vi "Get state -- subVI.vi"(7 "Instrument Channel":string, 8 "error in (no error)":errorcluster, 10 "Address":u8, 11 "Device state in":T2=enum."Configuration") -> (0 "error out":errorcluster, 2 "Controller state":T1, 3 "Device state out":T2)   [LabVIEW 2020, in "FCR100.lvlib"]
uses:
  FCR100.lvlib
  Device state -- enum.ctl
  Controller state -- enum.ctl
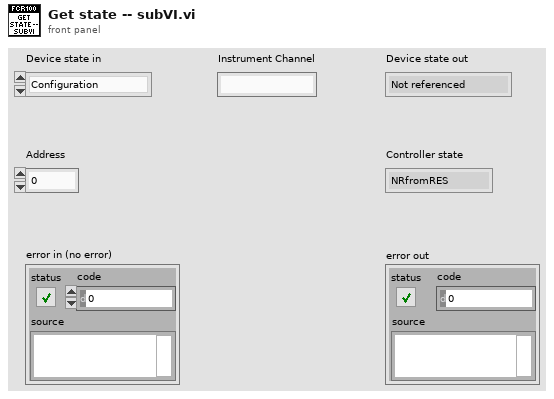
[diagram p1: front panel]
types:
  T1 = typedef "FCR100.lvlib/Controller state -- enum.ctl" = enum16{"NRfromRES", "NRfromHOM", "NRfromCONF", "NRfromDIS", "NRfromRDY", "NRfromMOV", "NR-NPM", "CONFIG", "HOMING", "MOVING", "RDYfromHOM", "RDYfromMOV", "RDYfromDIS", "DISfromRDY", "DISfromMOV"}
  T2 = typedef "FCR100.lvlib/Device state -- enum.ctl" = enum16{"Not referenced", "Configuration", "Disable", "Ready", "Homing", "Motion"}
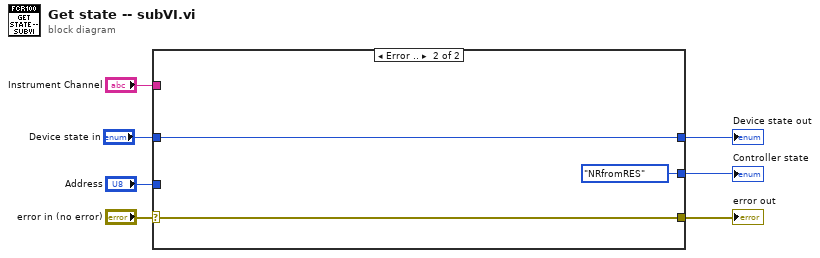
[diagram p0: block diagram]
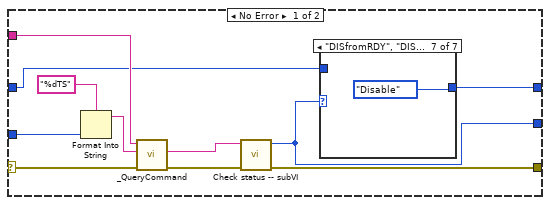
[diagram p2: hidden frame]
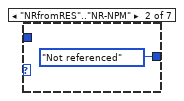
[diagram p4: hidden frame]
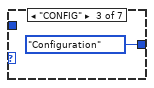
[diagram p5: hidden frame]
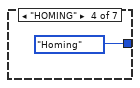
[diagram p6: hidden frame]
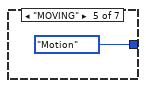
[diagram p7: hidden frame]
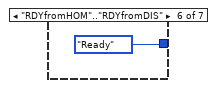
[diagram p8: hidden frame]
diagram:
  n1 = case shown="Error .." "error in (no error)" {
    selector: "error in (no error)" -> [w10 w28]
    tunnel: [w18 w28] -> w7
    tunnel: "Address" -> [w14 _]
    tunnel: "Instrument Channel" -> [w12 _]
    tunnel: "Device state in" -> [w11 w27]
    tunnel: [w9 w27] -> w2
    tunnel: [w8 Controller_state_--_enum."NRfromRES" ("Controller state")] -> w1
    frame No Error {
      n2 = Format Into String(format string="%dTS", w14) -> (resulting string=w16:string)  [unwired: 2 in, 1 out]
      n3 = call "_QueryCommand.vi"("error in"=w10, "Command"=w16, "Instrument Channel in"=w12) -> ("error out"=w17:errorcluster, "Response"=w13:string)  [unwired: 6 in, 1 out]
      n4 = call "Check status -- subVI.vi"("error in (no error)"=w17, "Input string"=w13) -> ("error out"=w18:errorcluster, "Controller state"=w8:T1)  [unwired: 8 in]
      n5 = case shown="\"DISfromRDY\", \"DISfromMOV\"" w8 {
        tunnel: [w19 Device_state_--_enum."Not referenced" ("Device state") Device_state_--_enum."Configuration" ("Device state") Device_state_--_enum."Homing" ("Device state") Device_state_--_enum."Motion" ("Device state") Device_state_--_enum."Ready" ("Device state") Device_state_--_enum."Disable" ("Device state")] -> w9
        tunnel: w11 -> [w19 _ _ _ _ _ _]
        frame Default {
        }
        frame "NRfromRES".."NR-NPM" {
        }
        frame "CONFIG" {
        }
        frame "HOMING" {
        }
        frame "MOVING" {
        }
        frame "RDYfromHOM".."RDYfromDIS" {
        }
        frame "DISfromRDY", "DISfromMOV" {
        }
      }
    }
    frame Error {
    }
  }
  "error out" <- w7
  "Device state out" <- w2
  "Controller state" <- w1
